vi "Memory.Pointer.New Subset Pointer.vi"(8 "error in (no error)":errorcluster, 9 "length":i64 format="%d bytes", 10 "offset":i64 format="%d bytes", 11 "Pointer in":refnum<class "Memory.Pointer.lvclass">) -> (0 "error out":errorcluster, 2 "subset Pointer":refnum<class "Memory.Pointer.lvclass">, 3 "Pointer out":refnum<class "Memory.Pointer.lvclass">)   [LabVIEW 2016, in "LabVIEW Memory Manager.lvlib" / "Memory.Pointer.lvclass"]
uses:
  Memory.Pointer.lvclass
  Memory.Pointer.lvclass/Memory.Pointer.ctl
  Accessors/Memory.Pointer.Set Address.vi
  Memory.Pointer.Offset to Address.Safe.vi
  Accessors/Memory.Pointer.Get Size.vi
  Memory.Pointer.Bounds Check.Length.vi
  Accessors/Memory.Pointer.Get Address.vi
  Memory.Pointer.Bounds Check.Offset.vi
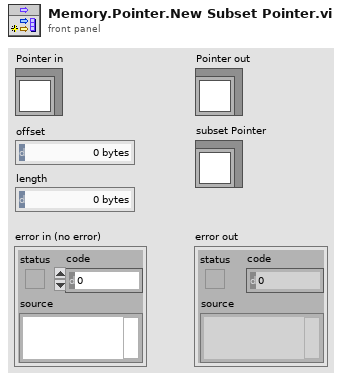
[diagram p1: front panel]
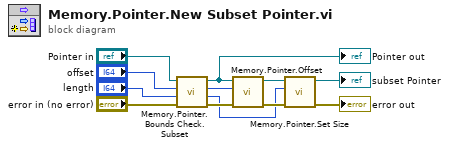
[diagram p0: block diagram]
diagram:
  n1 = call "Memory.Pointer.Bounds Check.Subset.vi"("error in (no error)"="error in (no error)", "length"="length", "offset"="offset", "Pointer in"="Pointer in") -> ("error out"=w12:errorcluster, "length out"=w1:i64, "offset out"=w6:i64, "Pointer out"=w7:refnum<class "Memory.Pointer.lvclass">)  [unwired: 3 in, 1 out]
  "Pointer out" <- w7
  n2 = call "Memory.Pointer.Offset.vi"("error in (no error)"=w12, "offset"=w6, "Pointer in"=w7) -> ("error out"=w4:errorcluster, "Pointer out"=w5:refnum<class "Memory.Pointer.lvclass">)  [unwired: 7 in]
  n3 = call "Memory.Pointer.Set Size.vi"("error in (no error)"=w4, "size"=w1, "Pointer in"=w5) -> ("error out"=→"error out":errorcluster, "Pointer out"=→"subset Pointer":refnum<class "Memory.Pointer.lvclass">)  [unwired: 7 in]
